vi "Format Complex Double Numeric Into String.vi"(0 "Complex Double Numeric":cdb, 1 "# of Significant Digits (17)":u8=17) -> (2 "Complex Double String":string)   [LabVIEW 2020]
doc: "This VI converts a complex double numeric value into a string. You may optionally supply the number of significant digits to record for the real and imaginary parts. This VI uses the %g format code to generate the string. See help for the Format Into String function for details."
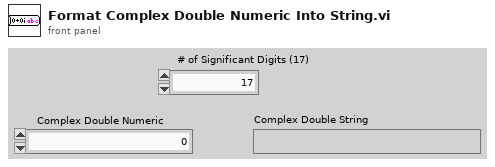
[diagram p1: front panel]
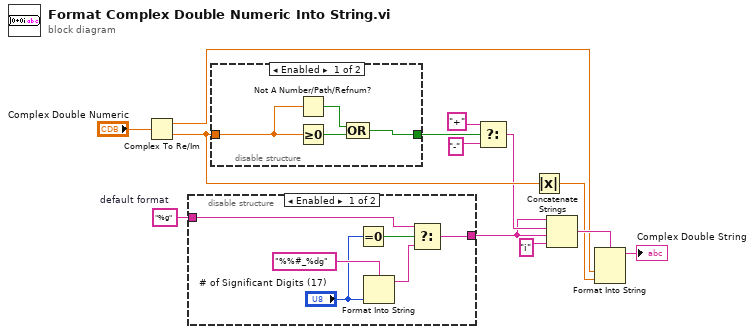
[diagram p0: block diagram]
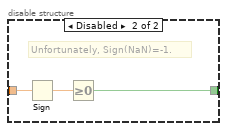
[diagram p2: hidden frame]
diagram:
  w3 = "%g"  # default format
  n1 = Complex To Re/Im(x + iy="Complex Double Numeric") -> (x=w6:dbl, y=w13:dbl)
  n2 = disable-structure shown="Enabled" {
    disable-tunnel: [w15 w20] -> w8
    disable-tunnel: w3 -> [w14 w20]
    frame Enabled {
      n3 = Equal To 0?(x="# of Significant Digits (17)") -> (x = 0?=w16:bool)
      n4 = Format Into String(format string="%%#_%dg", "# of Significant Digits (17)") -> (resulting string=w17:string)  [unwired: 2 in, 1 out]
      n5 = Select(t=w14, s=w16, f=w17) -> (s? t:f=w15:string)
    }
    frame Disabled {
    }
  }
  n6 = disable-structure shown="Enabled" {
    disable-tunnel: w13 -> [w22 w27]
    disable-tunnel: [w21 w25] -> w11
    frame Enabled {
      n7 = Not A Number/Path/Refnum?(number/path/refnum=w22) -> (NaN/Path/Refnum?=w24:bool)
      n8 = Greater Or Equal To 0?(x=w22) -> (x >= 0?=w23:bool)
      n9 = Compound Arithmetic op=OR(w24, w23) -> (w21:bool)
    }
    frame Disabled {
      # "Unfortunately, Sign(NaN)=-1."
      n10 = Sign(1:w27) -> (0:w26:dbl)
      n11 = Greater Or Equal To 0?(x=w26) -> (x >= 0?=w25:bool)
    }
  }
  n12 = Select(t="+", s=w11, f="-") -> (s? t:f=w9:string)
  n13 = Absolute Value(x=w13) -> (abs(x)=w5:dbl)
  n14 = Concatenate Strings(w8, w9, w8, "i" ("string")) -> (w7:string)
  n15 = Format Into String(format string=w7, w6, w5) -> (resulting string=→"Complex Double String":string)  [unwired: 2 in, 1 out]
